vi "Pasco_Harvester.vi"(11 "HarvClustIn":T1 {"HarvPOTElev" scale=0.0..5.0; "HarvManualElev" scale=-1.0..1.0; "HarvRollerBDesSpd" scale=-1.0..1.0; "HarvRollerFDesSpd" scale=-1.0..1.0}) -> (3 "HarvClustOut":T2 {"HarvOutRollerB" scale=-1.0..1.0; "HarvOutRollerF" scale=-1.0..1.0; "HarvOutElev" scale=-1.0..1.0})   [LabVIEW 2012]
panel:
  in  "HarvConstArrayElev":dbl[](array[numeric])
  in  "Harvester Speed Multiplier":dbl=0.75
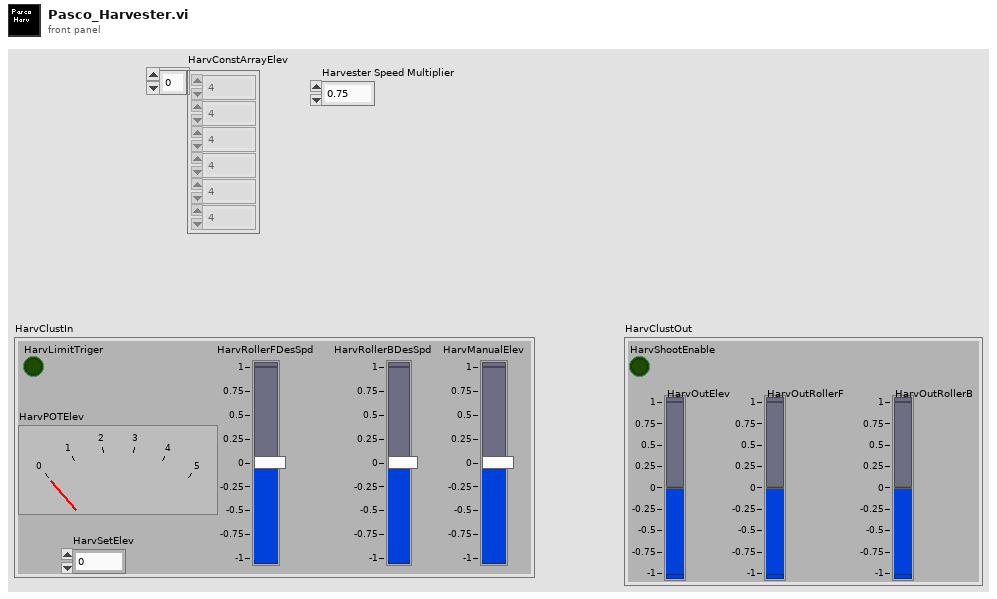
[diagram p1: front panel]
types:
  T1 = cluster{"HarvLimitTriger":bool, "HarvRollerFDesSpd":dbl, "HarvRollerBDesSpd":dbl, "HarvManualElev":dbl, "HarvPOTElev":dbl, "HarvSetElev":i32}
  T2 = cluster{"HarvOutElev":dbl, "HarvShootEnable":bool, "HarvOutRollerF":dbl, "HarvOutRollerB":dbl}
  T3 = cluster{"HarvOutElev":dbl, "HarvShootEnable":bool, "PWM Power":dbl, "PWM Power":dbl}
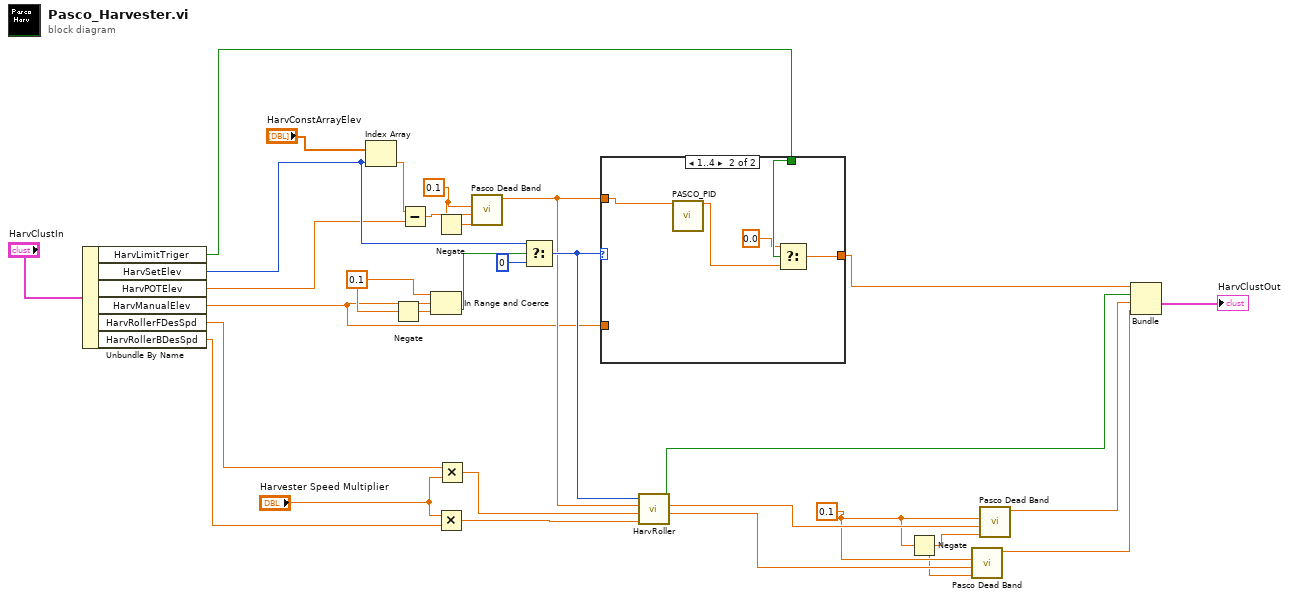
[diagram p0: block diagram]
diagram:
  w2 = 0.1 ("upper limit")
  w23 = 0.1 ("upper limit")
  w27 = 0.1 ("upper limit")
  n1 = Unbundle By Name("HarvClustIn") -> ("HarvLimitTriger"=w7:bool, "HarvSetElev"=w15:i32, "HarvPOTElev"=w14:dbl, "HarvManualElev"=w13:dbl, "HarvRollerFDesSpd"=w12:dbl, "HarvRollerBDesSpd"=w11:dbl)
  n2 = Index Array(array="HarvConstArrayElev", index=w15) -> (element=w30:dbl)
  n3 = Negate(x=w23) -> (-x=w24:dbl)
  n4 = Subtract(x=w30, y=w14) -> (x-y=w28:dbl)
  n5 = In Range and Coerce(upper limit=w23, x=w13, lower limit=w24) -> (In Range?=w22:bool)  [unwired: 1 out]
  n6 = Negate(x=w27) -> (-x=w26:dbl)
  n7 = Multiply(x="Harvester Speed Multiplier", y=w11) -> (x*y=w19:dbl)
  n8 = Multiply(x=w12, y="Harvester Speed Multiplier") -> (x*y=w20:dbl)
  n9 = call "Pasco Dead Band.vi"("lower limit"=w26, "PWM Power"=w28, "upper limit"=w27) -> ("PWM Power"=w17:dbl)  [unwired: 7 in, 1 out]
  n10 = Select(t=w15, s=w22, f=0) -> (s? t:f=w18:i32)
  n11 = case shown="1..4" w18 {
    tunnel: w17 -> [_ w36]
    tunnel: w13 -> [w31 _]
    tunnel: [w31 w35] -> w9
    tunnel: w7 -> [_ w33]
    frame 0, Default {
    }
    frame 1..4 {
      n12 = call "PASCO_PID.vi"("Delta"=w36) -> ("HarvOutElev"=w34:dbl)  [unwired: 14 in]
      n13 = Select(t=0.0, s=w33, f=w34) -> (s? t:f=w35:dbl)
    }
  }
  n14 = call "HarvRoller.vi"("HarvRollerBDesSpd"=w19, "HarvRollerFDesSpd"=w20, "HarvOutElev"=w17, "HarvSetElev"=w18) -> ("HarvOutRollerB"=w5:dbl, "HarvOutRollerF"=w6:dbl, "HarvShootEnable"=w8:bool)  [unwired: 5 in]
  n15 = Negate(x=w2) -> (-x=w1:dbl)
  n16 = call "Pasco Dead Band.vi"("lower limit"=w1, "PWM Power"=w5, "upper limit"=w2) -> ("PWM Power"=w4:dbl)  [unwired: 7 in, 1 out]
  n17 = call "Pasco Dead Band.vi"("lower limit"=w1, "PWM Power"=w6, "upper limit"=w2) -> ("PWM Power"=w3:dbl)  [unwired: 7 in, 1 out]
  n18 = Bundle("HarvOutElev"=w9, "HarvShootEnable"=w8, "PWM Power"=w3, "PWM Power"=w4) -> (→"HarvClustOut":T3)  [unwired: 1 in]
